vi "Extract Window Names.vi"(1 "window names":u8[](array[numeric])) -> (0 "application names":string[](array[string]))   [LabVIEW 2011]
doc: "This VI accepts an array of unsigned bytes and separates it into an array of strings. The string elements must be separated by double NULL characters."
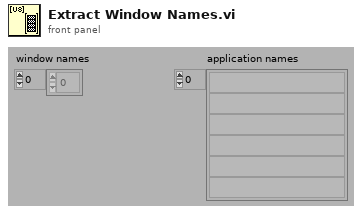
[diagram p1: front panel]
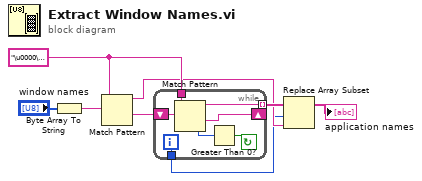
[diagram p0: block diagram]
diagram:
  w5 = "\u0000\u0000"
  n1 = Byte Array To String(unsigned byte array="window names") -> (string=w7:string)
  n2 = Match Pattern(string=w7, regular expression=w5) -> (before substring=w3:string, after substring=w6:string)  [unwired: 3 out]
  n3 = while {
    tunnel: [w9] -> w2
    tunnel: w5 -> [w11]
    tunnel: [w12] -> w4 mode=indexing
    shift-left: w6 -> [w15]
    shift-right: [w13] -> _
    i -> [w9]
    stop <- w10 continue-if-true
    n4 = Match Pattern(string=w15, regular expression=w11) -> (before substring=w12:string, after substring=w13:string, offset past match=w14:i32)  [unwired: 2 out]
    n5 = Greater Than 0?(x=w14) -> (x > 0?=w10:bool)
  }
  n6 = Replace Array Subset(array=w4, new element=w3, index=w2) -> (→"application names":string[])
